vi "IntegerMeasure.vi"(5 "EndTime":timestamp, 7 "StartTime":timestamp, 8 "error in":errorcluster, 11 "IntegerlMeasure":refnum<class "IntegerMeasure.lvclass">) -> (0 "error out":errorcluster, 3 "Passed":bool)   [LabVIEW 2020]
uses:
  <vilib>/Averna/ProligentResultProcessor/ProligentResultProcessor.lvlibp/Measure/IntegerMeasure/IntegerMeasure.lvclass
  C:/Program Files (x86)/National Instruments/LabVIEW 2020/vi.lib/Averna/ProligentResultProcessor/ProligentResultProcessor.lvlibp/Measure/Measure/Measure.lvclass
  <vilib>/Averna/ProligentResultProcessor/ProligentResultProcessor.lvlibp/Measure/IntegerMeasureLimit/IntegerMeasureLimit.lvclass
  C:/Program Files (x86)/National Instruments/LabVIEW 2020/vi.lib/Averna/ProligentResultProcessor/ProligentResultProcessor.lvlibp/Measure/RangeMeasureLimit/RangeMeasureLimit.lvclass
  C:/Program Files (x86)/National Instruments/LabVIEW 2020/vi.lib/Averna/ProligentResultProcessor/ProligentResultProcessor.lvlibp/Measure/MeasureLimit/MeasureLimit.lvclass
  <vilib>/Averna/ProligentResultProcessor/ProligentResultProcessor.lvlibp/Measure/RangeMeasureLimit/ComparisonType.ctl
  <vilib>/Averna/ProligentResultProcessor/ProligentResultProcessor.lvlibp/Measure/Measure/SetStartDate.vi
  <vilib>/Averna/ProligentResultProcessor/ProligentResultProcessor.lvlibp/Measure/Measure/SetMeasureExecutionStatus.vi
  <vilib>/Averna/ProligentResultProcessor/ProligentResultProcessor.lvlibp/Measure/IntegerMeasure/SetValue.vi
  <vilib>/Averna/ProligentResultProcessor/ProligentResultProcessor.lvlibp/Measure/Measure/SetComments.vi
  <vilib>/Averna/ProligentResultProcessor/ProligentResultProcessor.lvlibp/Measure/Measure/SetMeasureId.vi
  <vilib>/Averna/ProligentResultProcessor/ProligentResultProcessor.lvlibp/Measure/Measure/GetStartDate.vi
  <vilib>/Averna/ProligentResultProcessor/ProligentResultProcessor.lvlibp/Measure/Measure/GetMeasureExecutionStatus.vi
  <vilib>/Averna/ProligentResultProcessor/ProligentResultProcessor.lvlibp/Measure/IntegerMeasure/GetValue.vi
  <vilib>/Averna/ProligentResultProcessor/ProligentResultProcessor.lvlibp/Measure/Measure/GetComments.vi
  <vilib>/Averna/ProligentResultProcessor/ProligentResultProcessor.lvlibp/Measure/Measure/GetMeasureId.vi
  <vilib>/Averna/ProligentResultProcessor/ProligentResultProcessor.lvlibp/Measure/Measure/GetLimit.vi
  <vilib>/Averna/ProligentResultProcessor/ProligentResultProcessor.lvlibp/Measure/IntegerMeasureLimit/SetHigherBound.vi
  <vilib>/Averna/ProligentResultProcessor/ProligentResultProcessor.lvlibp/Measure/IntegerMeasureLimit/SetLowerBound.vi
  <vilib>/Averna/ProligentResultProcessor/ProligentResultProcessor.lvlibp/Measure/RangeMeasureLimit/GetComparisonType.vi
  <vilib>/Averna/ProligentResultProcessor/ProligentResultProcessor.lvlibp/Measure/IntegerMeasureLimit/GetHigherBound.vi
  <vilib>/Averna/ProligentResultProcessor/ProligentResultProcessor.lvlibp/Measure/IntegerMeasureLimit/GetLowerBound.vi
  <vilib>/Averna/ProligentResultProcessor/ProligentResultProcessor.lvlibp/Measure/MeasureLimit/GetLimitExpression.vi
  <vilib>/Averna/ProligentResultProcessor/ProligentResultProcessor.lvlibp/Measure/MeasureLimit/GetCustomData.vi
  <vilib>/Averna/ProligentResultProcessor/ProligentResultProcessor.lvlibp/Measure/Measure/GetCharacteristics.vi
  <vilib>/Averna/ProligentResultProcessor/ProligentResultProcessor.lvlibp/Measure/Measure/GetFailureReferences.vi
  <vilib>/Averna/ProligentResultProcessor/ProligentResultProcessor.lvlibp/Measure/Measure/GetCustomData.vi
  <vilib>/Averna/ProligentResultProcessor/ProligentResultProcessor.lvlibp/Measure/MeasureLimit/MeasureLimit.lvclass
  <vilib>/Averna/ProligentResultProcessor/ProligentResultProcessor.lvlibp/Model/CustomData/CustomData.lvclass
  <vilib>/Averna/ProligentResultProcessor/ProligentResultProcessor.lvlibp/Model/Characteristic/Characteristic.lvclass
  <vilib>/Averna/ProligentResultProcessor/ProligentResultProcessor.lvlibp/Failure/FailureReference/FailureReference.lvclass
  <vilib>/Averna/ProligentResultProcessor/ProligentResultProcessor.lvlibp/Measure/Measure/Measure.lvclass
  <vilib>/Averna/ProligentResultProcessor/ProligentResultProcessor.lvlibp/Measure/RangeMeasureLimit/RangeMeasureLimit.lvclass
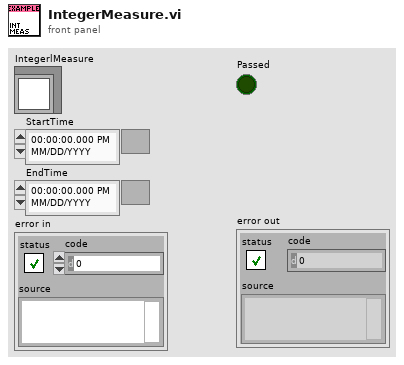
[diagram p1: front panel]
types:
  T1 = typedef "ProligentResultProcessor.lvlibp/RangeMeasureLimit.lvclass/ComparisonType.ctl" = enum16{"LowerBound <= X <= HigherBound", "LowerBound < X <= HigherBound", "LowerBound <= X < HigherBound", "LowerBound < X < HigherBound", "LowerBound <= X", "LowerBound < X", "X <= HigherBound", "X < HigherBound", "X == HigherBound", "X != HigherBound", "X <= LowerBound OR HigherBound <= X", "X < LowerBound OR HigherBound <= X", "X <= LowerBound OR HigherBound < X", "X < LowerBound OR HigherBound < X"}
  T2 = enum16{"PASS", "FAIL", "NOT_COMPLETED", "ABORTED"}
  T3 = enum16{"LowerBound <= X <= HigherBound", "LowerBound < X <= HigherBound", "LowerBound <= X < HigherBound", "LowerBound < X < HigherBound", "LowerBound <= X", "LowerBound < X", "X <= HigherBound", "X < HigherBound", "X == HigherBound", "X != HigherBound", "X <= LowerBound OR HigherBound <= X", "X < LowerBound OR HigherBound <= X", "X <= LowerBound OR HigherBound < X", "X < LowerBound OR HigherBound < X"}
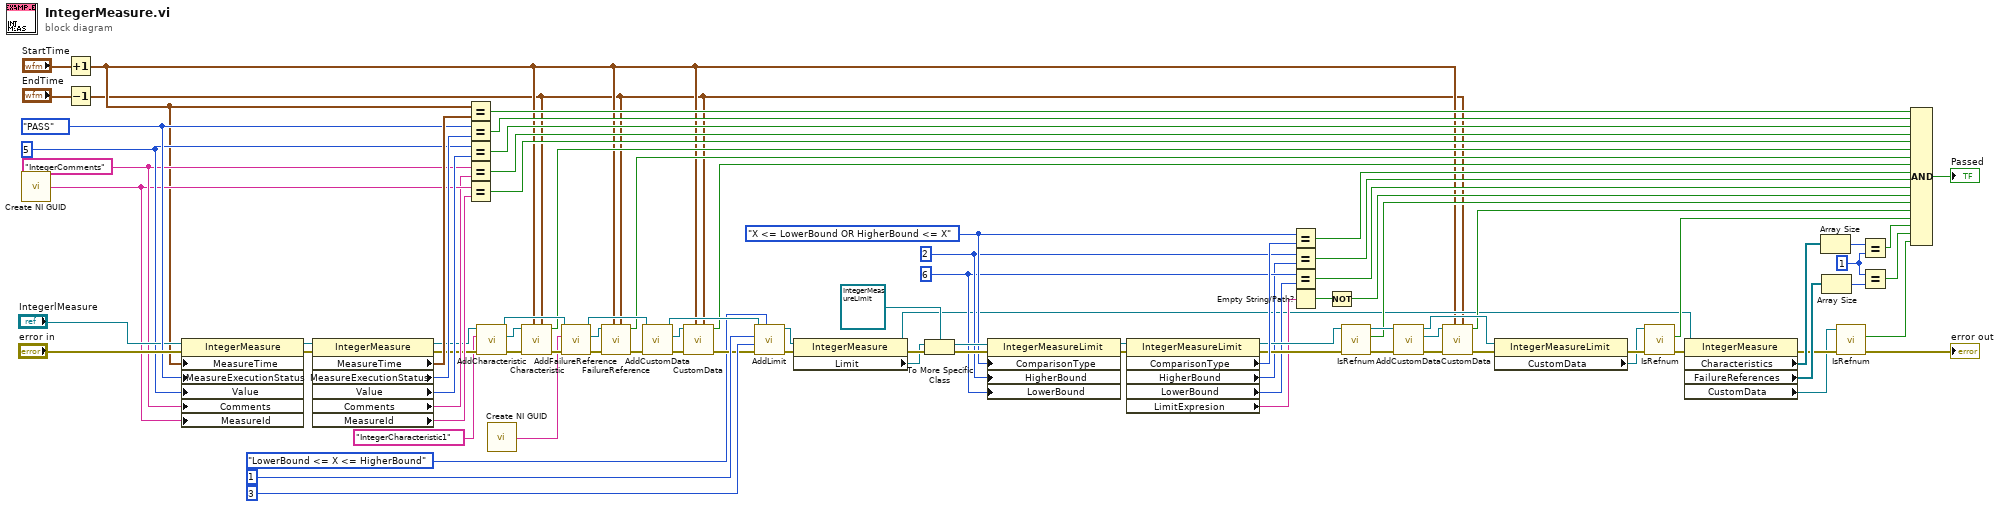
[diagram p0: block diagram]
diagram:
  w14 = 1
  w39 = "IntegerComments"
  w51 = i64 6 ("LowerBound")
  w52 = i64 2 ("LowerBound")
  w53 = ComparisonType."X <= LowerBound OR HigherBound <= X" ("ComparisonType")
  w44 = i64 5
  w80 = T2."PASS" ("ProcessRunStatus")
  n1 = call <vilib>:"Create NI GUID.vi"() -> ("NI GUID"=w38:string)
  n2 = Increment(x="StartTime") -> (x+1=w3:timestamp)
  n3 = Decrement(x="EndTime") -> (x-1=w2:timestamp)
  n4 = property class="IntegerMeasure"(reference="IntegerlMeasure", error in="error in", "MeasureTime"=w3, "MeasureExecutionStatus"=w80, "Value"=w44, "Comments"=w39, "MeasureId"=w38) -> (reference out=w91:refnum<class "IntegerMeasure.lvclass">, error out=w90:errorcluster)
  n5 = property class="IntegerMeasure"(reference=w91, error in=w90) -> (reference out=w23:refnum<class "IntegerMeasure.lvclass">, error out=w25:errorcluster, "MeasureTime"=w89:timestamp, "MeasureExecutionStatus"=w88:T2, "Value"=w87:i64, "Comments"=w37:string, "MeasureId"=w36:string)
  n6 = Equal?(x=w3, y=w89) -> (x = y?=w86:bool)
  n7 = Equal?(x=w80, y=w88) -> (x = y?=w85:bool)
  n8 = Equal?(x=w44, y=w87) -> (x = y?=w84:bool)
  n9 = Equal?(x=w39, y=w37) -> (x = y?=w41:bool)
  n10 = Equal?(x=w38, y=w36) -> (x = y?=w40:bool)
  n11 = call <vilib>:"AddCharacteristic.vi"("error in (no error)"=w25, "FullName"="IntegerCharacteristic1", "Measure in"=w23) -> ("error out"=w35:errorcluster, "Characteristic"=w34:refnum<class "Characteristic.lvclass">, "Measure out"=w32:refnum<class "IntegerMeasure.lvclass">)  [unwired: 6 in]
  n12 = call <vilib>:"Create NI GUID.vi"() -> ("NI GUID"=w4:string)
  n13 = call "Characteristic.vi"("EndTime"=w2, "StartTime"=w3, "error in (no error)"=w35, "Characteristic in"=w34) -> ("error out"=w33:errorcluster, "Passed"=w21:bool)  [unwired: 6 in]
  n14 = call <vilib>:"AddFailureReference.vi"("error in (no error)"=w33, "Id"=w4, "Measure in"=w32) -> ("error out"=w27:errorcluster, "FailureReference"=w26:refnum<class "FailureReference.lvclass">, "Measure out"=w29:refnum<class "IntegerMeasure.lvclass">)  [unwired: 6 in]
  n15 = call "FailureReference.vi"("EndTime"=w2, "StartTime"=w3, "error in"=w27, "FailureReference"=w26) -> ("error out"=w31:errorcluster, "Passed"=w20:bool)  [unwired: 6 in]
  n16 = call <vilib>:"AddCustomData.vi"("error in (no error)"=w31, "Measure in"=w29) -> ("error out"=w30:errorcluster, "CustomData"=w28:refnum<class "CustomData.lvclass">, "Measure out"=w22:refnum<class "IntegerMeasure.lvclass">)  [unwired: 7 in]
  n17 = call "CustomData.vi"("EndTime"=w2, "StartTime"=w3, "error in"=w30, "CustomData"=w28) -> ("error out"=w24:errorcluster, "Passed"=w19:bool)  [unwired: 6 in]
  n18 = call <vilib>:"AddLimit.vi"("ComparisonType"=ComparisonType."LowerBound <= X <= HigherBound", "error in"=w24, "HigherBond"=i64 3 ("LowerBound"), "LowerBound"=i64 1, "IntergerMeasure in"=w22) -> ("error out"=w74:errorcluster, "IntergerMeasure out"=w79:refnum<class "IntegerMeasure.lvclass">)  [unwired: 4 in, 1 out]
  n19 = property class="IntegerMeasure"(reference=w79, error in=w74) -> (reference out=w17:refnum<class "IntegerMeasure.lvclass">, error out=w78:errorcluster, "Limit"=w75:refnum<class "MeasureLimit.lvclass">)
  n20 = To More Specific Class(target class=refnum<class "IntegerMeasureLimit.lvclass"> refnum ("ProligentResultProcessor:IntegerMeasureLimit"), reference=w75, error in=w78) -> (specific class reference=w76:refnum<class "IntegerMeasureLimit.lvclass">, error out=w77:errorcluster)
  n21 = property class="IntegerMeasureLimit"(reference=w76, error in=w77, "ComparisonType"=w53, "HigherBound"=w52, "LowerBound"=w51) -> (reference out=w73:refnum<class "IntegerMeasureLimit.lvclass">, error out=w72:errorcluster)
  n22 = property class="IntegerMeasureLimit"(reference=w73, error in=w72) -> (reference out=w64:refnum<class "IntegerMeasureLimit.lvclass">, error out=w69:errorcluster, "ComparisonType"=w71:T3, "HigherBound"=w50:i64, "LowerBound"=w49:i64, "LimitExpresion"=w54:string)
  n23 = Equal?(x=w53, y=w71) -> (x = y?=w48:bool)
  n24 = Equal?(x=w52, y=w50) -> (x = y?=w47:bool)
  n25 = Equal?(x=w51, y=w49) -> (x = y?=w46:bool)
  n26 = Empty String/Path?(string/path=w54) -> (empty?=w70:bool)
  n27 = Not(x=w70) -> (.not. x?=w42:bool)
  n28 = call <vilib>:"IsRefnum.vi"("error in"=w69, "MeasureLimit in"=w64) -> ("error out"=w65:errorcluster, "IsRefnum"=w62:bool, "MeasureLimit out"=w63:refnum<class "IntegerMeasureLimit.lvclass">)  [unwired: 7 in]
  n29 = call <vilib>:"AddCustomData.vi"("error in"=w65, "MeasureLimit in"=w63) -> ("error out"=w60:errorcluster, "CustomData"=w58:refnum<class "CustomData.lvclass">, "MeasureLimit out"=w61:refnum<class "IntegerMeasureLimit.lvclass">)  [unwired: 7 in]
  n30 = call "CustomData.vi"("EndTime"=w2, "StartTime"=w3, "error in"=w60, "CustomData"=w58) -> ("error out"=w59:errorcluster, "Passed"=w57:bool)  [unwired: 6 in]
  n31 = property class="IntegerMeasureLimit"(reference=w61, error in=w59) -> (error out=w68:errorcluster, "CustomData"=w67:refnum<class "CustomData.lvclass">)  [unwired: 1 out]
  n32 = call <vilib>:"IsRefnum.vi"("error in"=w68, "CustomDataType in"=w67) -> ("error out"=w18:errorcluster, "IsRefnum"=w66:bool)  [unwired: 7 in, 1 out]
  n33 = property class="IntegerMeasure"(reference=w17, error in=w18) -> (error out=w9:errorcluster, "Characteristics"=w11:refnum<class "Characteristic.lvclass">[], "FailureReferences"=w10:refnum<class "FailureReference.lvclass">[], "CustomData"=w7:refnum<class "CustomData.lvclass">)  [unwired: 1 out]
  n34 = Array Size(array=w11) -> (size(s)=w16:i32)
  n35 = Array Size(array=w10) -> (size(s)=w15:i32)
  n36 = call <vilib>:"IsRefnum.vi"("error in"=w9, "CustomDataType in"=w7) -> ("error out"=→"error out":errorcluster, "IsRefnum"=w6:bool)  [unwired: 7 in, 1 out]
  n37 = Equal?(x=w16, y=w14) -> (x = y?=w13:bool)
  n38 = Equal?(x=w14, y=w15) -> (x = y?=w12:bool)
  n39 = Compound Arithmetic op=AND(w86, w85, w84, w41, w40, w21, w20, w19, w48, w47, w46, w42, w62, w57, w66, w13, w12, w6) -> (→"Passed":bool)
